vi "Create.vi"(7 "buffer size (10)":i32=10, 8 "error in (no error)":errorcluster, 11 "Ctrl Val.Set All":T1[](array[typedef])) -> (0 "error out":errorcluster, 3 "UndoObject out":refnum<class "UndoObject.lvclass">)   [LabVIEW 2015, in "UndoLibrary.lvlib" / "UndoObject.lvclass"]
doc: "This VI creates the references to store the values of the controls."
uses:
  UndoObject.lvclass
  Support VIs/DataClass/Controls/cluster_Control Value.ctl
  Support VIs/DataClass/DataObject.lvclass
  Support VIs/DataClass/DataObject.lvclass/DataObject.ctl
  UndoObject.lvclass/UndoObject.ctl
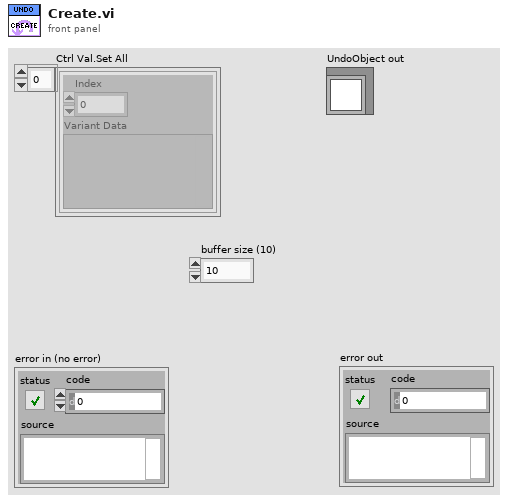
[diagram p1: front panel]
types:
  T1 = typedef "UndoLibrary.lvlib/DataObject.lvclass/cluster_Control Value.ctl" = cluster{"Index":i32, "Variant Data":variant}
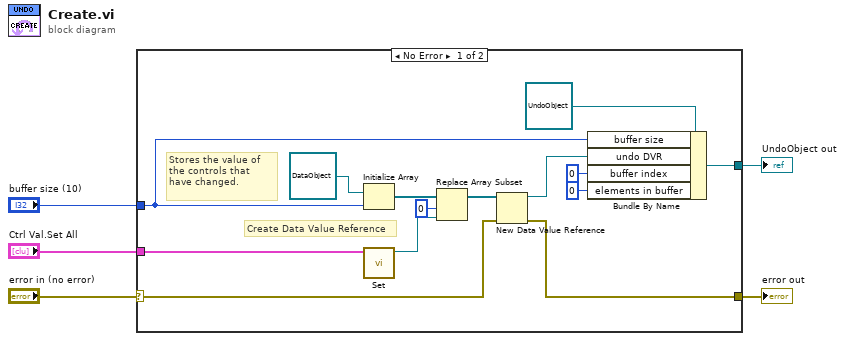
[diagram p0: block diagram]
diagram:
  n1 = case shown="No Error" "error in (no error)" {
    selector: "error in (no error)" -> [w16 w20]
    tunnel: "Ctrl Val.Set All" -> [w10 _]
    tunnel: "buffer size (10)" -> [w13 _]
    tunnel: [w18 _] -> w1
    tunnel: [w15 w20] -> w2
    frame No Error {
      # "Stores the value of the controls that have changed."
      # "Create Data Value Reference"
      n2 = Initialize Array(refnum<class "DataObject.lvclass"> refnum ("UndoLibrary.lvlib:DataObject.lvclass"), w13) -> (w9:refnum<class "DataObject.lvclass">[])
      n3 = call "Set.vi"("Conrol Value[]"=w10) -> ("DataObject out"=w7:refnum<class "DataObject.lvclass">)  [unwired: 9 in, 1 out]
      n4 = Replace Array Subset(array=w9, new element=w7, index=0) -> (w8:refnum<class "DataObject.lvclass">[])
      n5 = New Data Value Reference(data value=w8, error in=w16) -> (data value reference=w14:refnum<data-value>, error out=w15:errorcluster)
      n6 = Bundle By Name(cluster=refnum<class "UndoObject.lvclass"> refnum ("UndoLibrary.lvlib:UndoObject.lvclass"), "buffer size"=w13, "undo DVR"=w14, "buffer index"=0, "elements in buffer"=0) -> (w18:refnum<class "UndoObject.lvclass">)
    }
    frame Error {
    }
  }
  "error out" <- w2
  "UndoObject out" <- w1
